vi "set_x_fractions.vi"(6 "x scan segment fraction":dbl, 8 "error in (no error)":errorcluster, 9 "x offset fly back fraction":dbl, 10 "x offset fly forward fraction":dbl, 11 "TrajectoryAK101022Resonance in":refnum<class "TrajectoryAK101022Resonance.lvclass">) -> (0 "error out":errorcluster, 3 "TrajectoryAK101022Resonance out":refnum<class "TrajectoryAK101022Resonance.lvclass">)   [LabVIEW 2010, in "TrajectoryAK101022Resonance.lvclass"]
uses:
  TrajectoryAK101022Resonance.lvclass
  TrajectoryAK101022Resonance.lvclass/TrajectoryAK101022Resonance.ctl
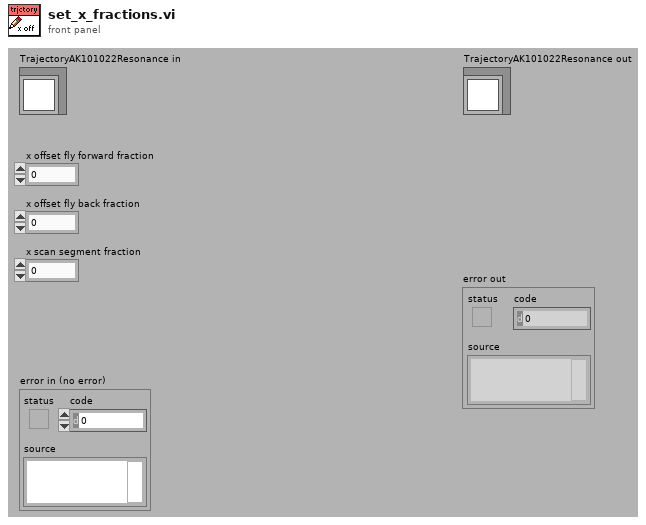
[diagram p1: front panel]
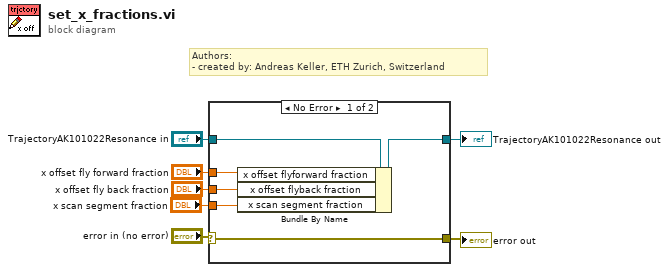
[diagram p0: block diagram]
diagram:
  # "Authors: \n- created by: Andreas Keller, ETH Zurich, Switzerland"
  n1 = case shown="No Error" "error in (no error)" {
    selector: "error in (no error)" -> [w13 w15]
    tunnel: [w13 w15] -> w6
    tunnel: "TrajectoryAK101022Resonance in" -> [w11 w14]
    tunnel: [w12 w14] -> w4
    tunnel: "x offset fly forward fraction" -> [w10 _]
    tunnel: "x offset fly back fraction" -> [w9 _]
    tunnel: "x scan segment fraction" -> [w8 _]
    frame No Error {
      n2 = Bundle By Name(cluster=w11, "x offset flyforward fraction"=w10, "x offset flyback fraction"=w9, "x scan segment fraction"=w8) -> (w12:refnum<class "TrajectoryAK101022Resonance.lvclass">)
    }
    frame Error {
    }
  }
  "TrajectoryAK101022Resonance out" <- w4
  "error out" <- w6
